vi "Ch_setup_string.vi"(6 "Ch & spans":T1[](array[typedef]) {"low limit (-10V)" format="%.3f"; "high limit (10V)" format="%.3f"}) -> (1 "Output string":string)   [LabVIEW 2013]
uses:
  Controls/Ch_and_Spans.ctl
  Globals/Meas_global.vi
panel:
  out "length":i32
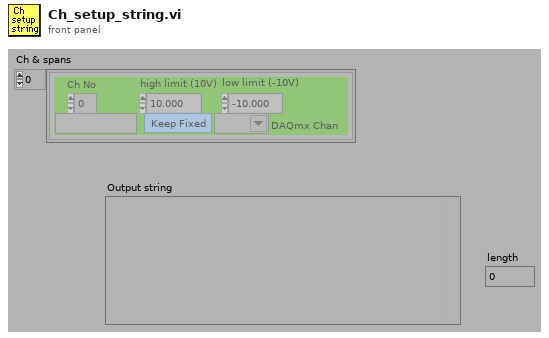
[diagram p1: front panel]
types:
  T1 = typedef "Ch_and_Spans.ctl" = cluster{"high limit (10V)":sgl, "low limit (-10V)":sgl, "Ch No":i16, "Var name":string, "Use Latest Calib":bool, "DAQmx Chan":tag}
  T2 = typedef "Analysis_info_cluster.ctl" = cluster{"Colour":u32, "Inst type":T3, "Inst name":string, "Symbol":string, "Code name":string, "Extra Info":string, "Inst Array":T4, "Extra Titles":string[], "Extra Values":string[], "U":dbl, "u^2":dbl, "u^3":dbl, "u^4":dbl, "Skew_u":dbl, "Kurt_u":dbl, "Sd Error in Mean":dbl, "% u'/U":dbl, "X":dbl, "Y":dbl, "Z":dbl, "Timescale integral to 25%":dbl, "Sd Error in Variance":dbl, "Calib File":path, "Calib Constants":dbl[], "Output Position":bool, "Full Stats":bool, "Av Sampling Rate":dbl, "Av No of Samples":dbl, "Total Meas Time (s)":dbl, "ADAM Ch Name":string}
  T3 = typedef "Inst_type.ctl" = enum16{"Propeller anemometer", "Raw voltage", "Pressure Transducer", "Pitot-static tube", "Preston tube", "Hot wire", "Cross wire 1", "Cross wire 2", "Generic Linear", "Generic Polynomial", "Generic BackPoly", "Fast FID", "Thermocouple", "Cold wire", "Pulsed Wire", "LDA Vel", "LDA Tran time", "LDA Arr time"}
  T4 = typedef "Instrument_Array.ctl" = enum16{"PWA", "LDA", "Analogue"}
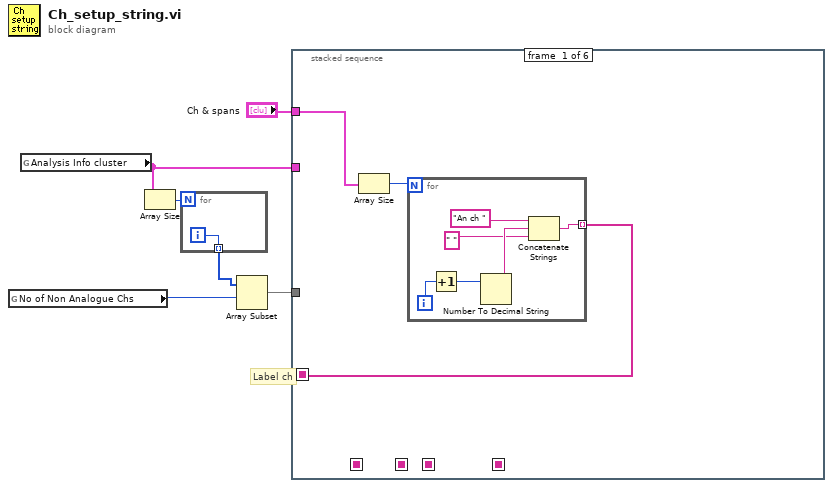
[diagram p0: block diagram]
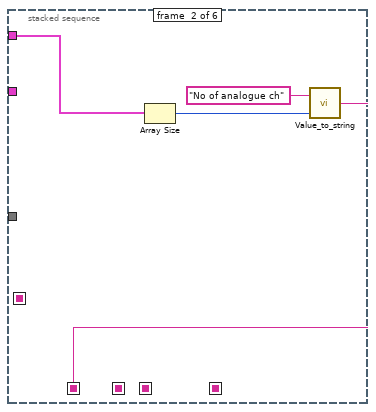
[diagram p2: hidden frame]
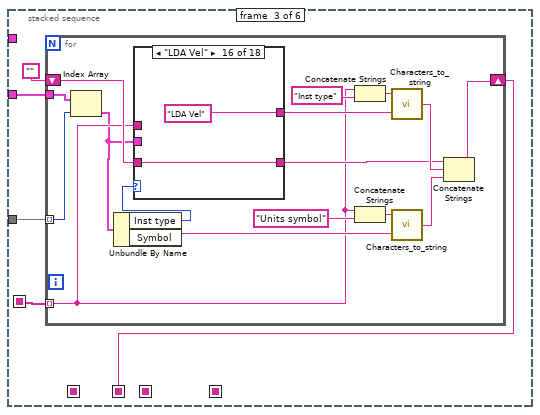
[diagram p3: hidden frame]
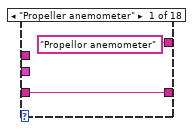
[diagram p4: hidden frame]
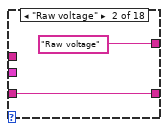
[diagram p5: hidden frame]
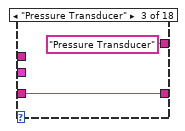
[diagram p6: hidden frame]
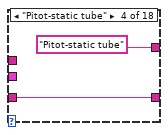
[diagram p7: hidden frame]
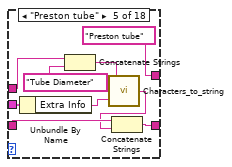
[diagram p8: hidden frame]
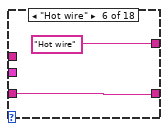
[diagram p9: hidden frame]
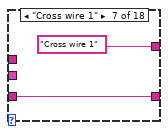
[diagram p10: hidden frame]
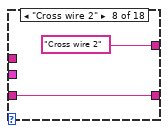
[diagram p11: hidden frame]
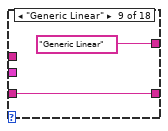
[diagram p12: hidden frame]
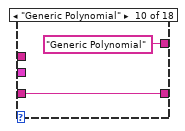
[diagram p13: hidden frame]
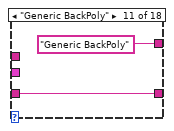
[diagram p14: hidden frame]
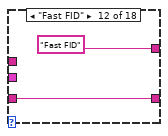
[diagram p15: hidden frame]
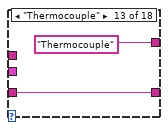
[diagram p16: hidden frame]
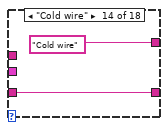
[diagram p17: hidden frame]
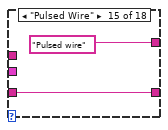
[diagram p18: hidden frame]
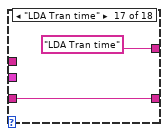
[diagram p19: hidden frame]
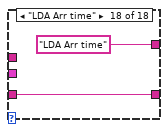
[diagram p20: hidden frame]
diagram:
  # "Label ch"
  n1 = global read "Meas_global.vi" "No of Non Analogue Chs"() -> (w2:i32)
  n2 = global read "Meas_global.vi" "Analysis Info cluster"() -> (w5:T2[])
  n3 = Array Size(array=w5) -> (size(s)=w4:i32)
  n4 = for {
    N: w4 -> [_]
    tunnel: [w7] -> w3 mode=indexing
    i -> [w7]
  }
  n5 = Array Subset(array=w3, index=w2) -> (w1:i32[])  [unwired: 1 in]
  n6 = stacked-sequence {
    seq-local: [_ _ w24 _ _ _] -> [_ _ _ _ _ w137]
    seq-local: [_ _ _ _ w118 _] -> [_ _ _ _ _ w136]
    seq-local: [w9 _ _ _ _ _] -> [_ _ w23 w87 w119 _]
    seq-local: [_ w17 _ _ _ _] -> [_ _ _ _ _ w133]
    seq-local: [_ _ _ w86 _ _] -> [_ _ _ _ _ w132]
    tunnel: "Ch & spans" -> [w8 w18 _ w85 _ _]
    tunnel: w5 -> [_ _ w22 _ w117 _]
    tunnel: w1 -> [_ _ w21 _ w116 _]
    frame #0 {
      n7 = Array Size(array=w8) -> (size(s)=w10:i32)
      n8 = for {
        N: w10 -> [_]
        tunnel: [w12] -> w9 mode=indexing
        i -> [w14]
        n9 = Increment(x=w14) -> (x+1=w13:i32)
        n10 = Number To Decimal String(number=w13) -> (decimal integer string=w16:string)  [unwired: 1 out]
        n11 = Concatenate Strings("An ch ", w16, " ") -> (w12:string)
      }
    }
    frame #1 {
      n12 = Array Size(array=w18) -> (size(s)=w19:i32)
      n13 = call "Value_to_string.vi"("Value"=w19, "Label for value"="No of analogue ch") -> ("Output string"=w17:string)  [unwired: 1 in]
    }
    frame #2 {
      n14 = for {
        shift-right: [w41] -> w24
        shift-left: "" -> [w32]
        tunnel: w23 -> [w29] mode=indexing
        tunnel: w22 -> [w28]
        tunnel: w21 -> [w27] mode=indexing
        n15 = Index Array(array=w28, index=w27) -> (element=w26:T2)
        n16 = Unbundle By Name(w26) -> ("Inst type"=w30:T3, "Symbol"=w40:string)
        n17 = case shown="\"LDA Vel\"" w30 {
          tunnel: ["Propellor anemometer" "Raw voltage" "Pressure Transducer" "Pitot-static tube" "Preston tube" "Hot wire" "Cross wire 1" "Cross wire 2" "Generic Linear" "Generic Polynomial" "Generic BackPoly" "Fast FID" "Thermocouple" "Cold wire" "Pulsed wire" "LDA Vel" "LDA Tran time" "LDA Arr time"] -> w39
          tunnel: w32 -> [w42 w44 w46 w48 w56 w59 w61 w63 w65 w67 w69 w71 w73 w75 w77 w79 w81 w83]
          tunnel: [w42 w44 w46 w48 w55 w59 w61 w63 w65 w67 w69 w71 w73 w75 w77 w79 w81 w83] -> w31
          tunnel: w26 -> [_ _ _ _ w58 _ _ _ _ _ _ _ _ _ _ _ _ _]
          tunnel: w29 -> [_ _ _ _ w51 _ _ _ _ _ _ _ _ _ _ _ _ _]
          frame "Propeller anemometer" {
          }
          frame "Raw voltage" {
          }
          frame "Pressure Transducer" {
          }
          frame "Pitot-static tube" {
          }
          frame "Preston tube" {
            n18 = Unbundle By Name(w58) -> ("Extra Info"=w57:string)
            n19 = Concatenate Strings(w51, "Tube Diameter") -> (w50:string)
            n20 = call "Characters_to_string.vi"("Characters to write"=w57, "Label for characters"=w50) -> ("Output string"=w53:string)
            n21 = Concatenate Strings(w56, w53) -> (w55:string)
          }
          frame "Hot wire" {
          }
          frame "Cross wire 1" {
          }
          frame "Cross wire 2" {
          }
          frame "Generic Linear" {
          }
          frame "Generic Polynomial" {
          }
          frame "Generic BackPoly" {
          }
          frame "Fast FID" {
          }
          frame "Thermocouple" {
          }
          frame "Cold wire" {
          }
          frame "Pulsed Wire" {
          }
          frame "LDA Vel" {
          }
          frame "LDA Tran time" {
          }
          frame "LDA Arr time" {
          }
        }
        n22 = Concatenate Strings(w29, "Inst type") -> (w33:string)
        n23 = Concatenate Strings(w29, "Units symbol") -> (w34:string)
        n24 = call "Characters_to_string.vi"("Characters to write"=w39, "Label for characters"=w33) -> ("Output string"=w35:string)
        n25 = call "Characters_to_string.vi"("Characters to write"=w40, "Label for characters"=w34) -> ("Output string"=w36:string)
        n26 = Concatenate Strings(w31, w35, w36) -> (w41:string)
      }
    }
    frame #3 {
      n27 = for {
        shift-right: [w114] -> w86
        shift-left: "" -> [w115]
        tunnel: w87 -> [w93] mode=indexing
        tunnel: w85 -> [w97] mode=indexing
        n28 = Unbundle By Name(w97) -> ("high limit (10V)"=w103:sgl, "low limit (-10V)"=w104:sgl, "Ch No"=w105:i16, "Use Latest Calib"=w96:bool, "DAQmx Chan"=w91:tag)
        n29 = Select(t="TRUE", s=w96, f="FALSE") -> (s? t:f=w98:string)
        n30 = Concatenate Strings(w93, "Use latest Calib") -> (w101:string)
        n31 = Concatenate Strings(w93, "High limit") -> (w111:string)
        n32 = Concatenate Strings(w93, "Low limit") -> (w110:string)
        n33 = Concatenate Strings(w93, "Ch No") -> (w107:string)
        n34 = Concatenate Strings(w93, "DAQ Ch") -> (w94:string)
        n35 = call "Value_to_string.vi"("Value"=w103, "Label for value"=w111) -> ("Output string"=w112:string)  [unwired: 1 in]
        n36 = call "Value_to_string.vi"("Value"=w104, "Label for value"=w110) -> ("Output string"=w106:string)  [unwired: 1 in]
        n37 = call "Value_to_string.vi"("Value"=w105, "Label for value"=w107) -> ("Output string"=w95:string)  [unwired: 1 in]
        n38 = call "Characters_to_string.vi"("Characters to write"=w91, "Label for characters"=w94) -> ("Output string"=w89:string)
        n39 = call "Characters_to_string.vi"("Characters to write"=w98, "Label for characters"=w101) -> ("Output string"=w90:string)
        n40 = Concatenate Strings(w115, w112, w106, w95, w89, w90) -> (w114:string)
      }
    }
    frame #4 {
      n41 = for {
        shift-right: [w130] -> w118
        shift-left: "" -> [w131]
        tunnel: w119 -> [w126] mode=indexing
        tunnel: w117 -> [w123]
        tunnel: w116 -> [w122] mode=indexing
        n42 = Index Array(array=w123, index=w122) -> (element=w121:T2)
        n43 = Unbundle By Name(w121) -> ("Calib File"=w124:path)
        n44 = Path To String(path=w124) -> (string=w125:string)
        n45 = Concatenate Strings(w126, "Calib filename") -> (w127:string)
        n46 = call "Characters_to_string.vi"("Characters to write"=w125, "Label for characters"=w127) -> ("Output string"=w128:string)
        n47 = Concatenate Strings(w131, w128) -> (w130:string)
      }
    }
    frame #5 {
      n48 = Concatenate Strings(w133, w137, w136, w132) -> (w134:string)
      "Output string" <- w134
      n49 = String Length(string=w134) -> (length=→"length":i32)
    }
  }
